vi "Write last phase.vi"(8 "error in (no error)":errorcluster, 10 "last phase":dbl[](array[numeric]), 11 "ScopeBase in":refnum<class "ScopeBase.lvclass">) -> (0 "error out":errorcluster, 3 "ScopeBase out":refnum<class "ScopeBase.lvclass">)   [LabVIEW 2018, in "ScopeBase.lvclass"]
uses:
  ScopeBase.lvclass
  ScopeBase.lvclass/ScopeBase.ctl
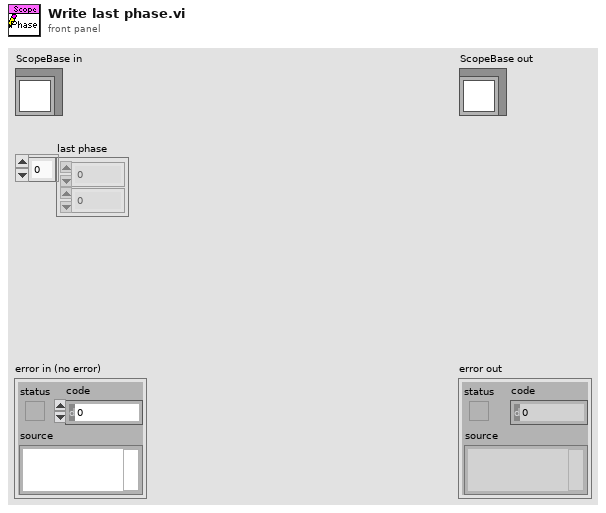
[diagram p1: front panel]
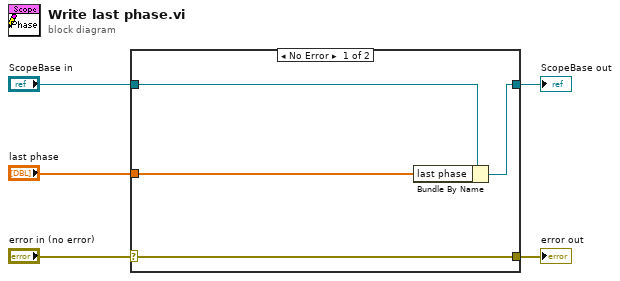
[diagram p0: block diagram]
diagram:
  n1 = case shown="No Error" "error in (no error)" {
    selector: "error in (no error)" -> [w9 w10]
    tunnel: [w9 w10] -> w4
    tunnel: [w7 w11] -> w2
    tunnel: "ScopeBase in" -> [w8 w11]
    tunnel: "last phase" -> [w6 _]
    frame No Error {
      n2 = Bundle By Name(cluster=w8, "last phase"=w6) -> (w7:refnum<class "ScopeBase.lvclass">)
    }
    frame Error {
    }
  }
  "error out" <- w4
  "ScopeBase out" <- w2
